vi "Add Routing Channel Folder.vi"(8 "error in":errorcluster, 9 "description":string, 10 "folder name":string, 11 "section in":T1 format="%.0x") -> (0 "error out":errorcluster, 2 "routing channel folder":T1 format="%.0x", 3 "section out":T1 format="%.0x")   [LabVIEW 2017, in "Routing and Faulting Scripting.lvlib"]
doc: "Creates and adds a routing channel with the specified configuration to the custom device."
uses:
  Routing and Faulting Scripting.lvlib
  <vilib>/NI Veristand/Custom Device API/Custom Device Item Ref.ctl
  Shared/Constants.vi
  <vilib>/NI Veristand/Custom Device API/Custom Device API.lvlib
  Shared/Routing and Faulting Shared.lvlib
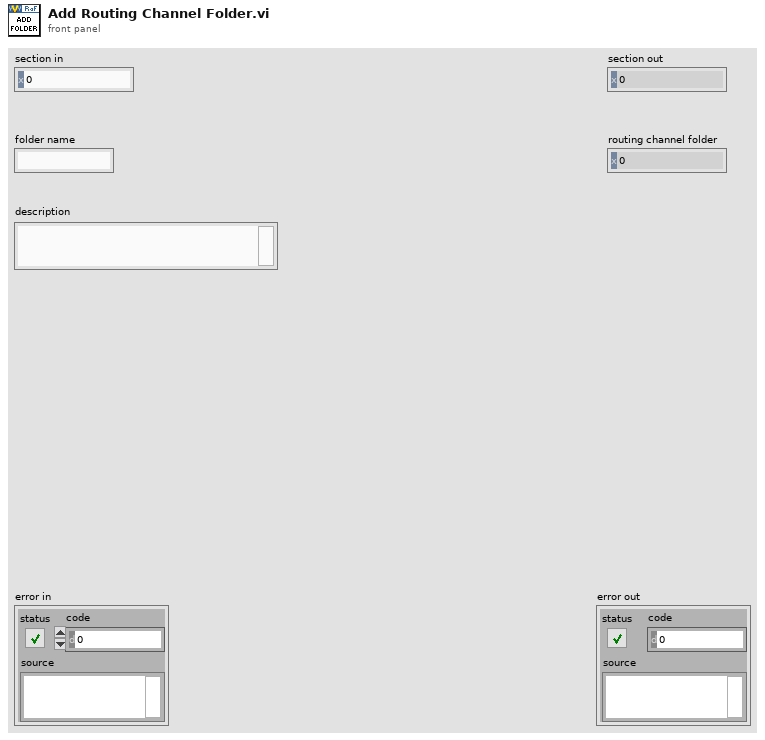
[diagram p1: front panel]
types:
  T1 = typedef "Custom Device API.lvlib/Custom Device Item Ref.ctl" = u64
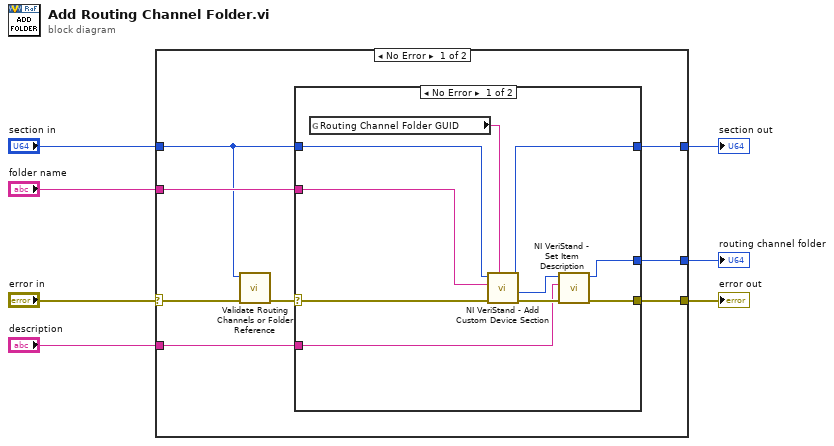
[diagram p0: block diagram]
diagram:
  n1 = case shown="No Error" "error in" {
    selector: "error in" -> [w10 w29]
    tunnel: [w13 w29] -> w7
    tunnel: [w15 w28] -> w6
    tunnel: "section in" -> [w8 w28]
    tunnel: "folder name" -> [w11 _]
    tunnel: [w12 _] -> w2
    tunnel: "description" -> [w14 _]
    frame No Error {
      n2 = call "Validate Routing Channels or Folder Reference.vi"("error in"=w10, "routing channels in"=w8) -> ("error out"=w9:errorcluster)  [unwired: 8 in, 1 out]
      n3 = case shown="No Error" w9 {
        selector: w9 -> [w16 w26]
        tunnel: w11 -> [w25 _]
        tunnel: w8 -> [w24 w27]
        tunnel: [w23 w27] -> w15
        tunnel: w14 -> [w21 _]
        tunnel: [w19 w26] -> w13
        tunnel: [w18 _] -> w12
        frame No Error {
          n4 = global read "Constants.vi" "Routing Channel Folder GUID"() -> (w17:string)
          n5 = call <vilib>:"NI VeriStand - Add Custom Device Section.vi"("GUID (Default Section)"=w17, "error in (no error)"=w16, "Section Name"=w25, "Parent Ref in"=w24) -> ("error out"=w22:errorcluster, "Section Ptr"=w20:T1, "Parent Ref out"=w23:T1)  [unwired: 4 in, 1 out]
          n6 = call <vilib>:"NI VeriStand - Set Item Description.vi"("error in (no error)"=w22, "Description"=w21, "Item Ref in"=w20) -> ("error out"=w19:errorcluster, "Item Ref out"=w18:T1)  [unwired: 6 in, 1 out]
        }
        frame Error {
        }
      }
    }
    frame Error {
    }
  }
  "error out" <- w7
  "section out" <- w6
  "routing channel folder" <- w2
